vi "Calculator.vi"() -> ()   [LabVIEW 2020]
panel:
  in  "Operator":T1(ring)
  out "Result":dbl
  in  "Input B":dbl
  in  "Input A":dbl
  # "Simple Calculator"
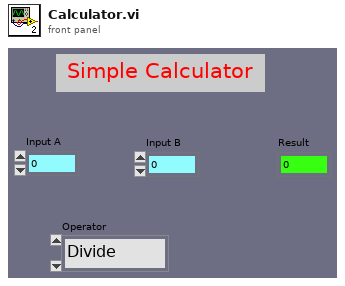
[diagram p1: front panel]
types:
  T1 = enum16{"Divide", "Multiply", "Add", "Subtract", ""}
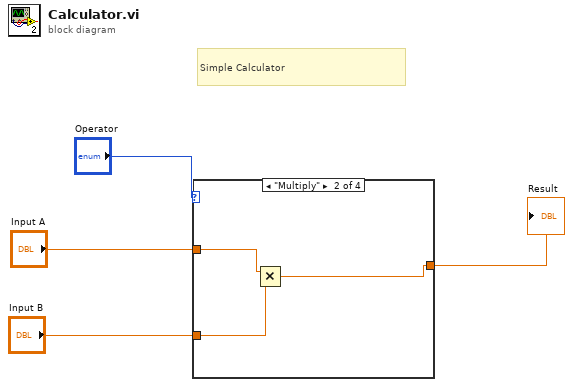
[diagram p0: block diagram]
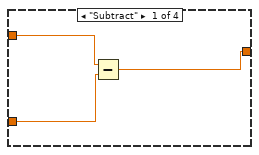
[diagram p2: hidden frame]
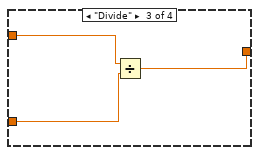
[diagram p3: hidden frame]
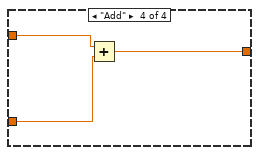
[diagram p4: hidden frame]
diagram:
  # "Simple Calculator"
  n1 = case shown="\"Multiply\"" "Operator" {
    tunnel: "Input A" -> [w7 w10 w13 w16]
    tunnel: "Input B" -> [w6 w9 w12 w15]
    tunnel: [w5 w8 w11 w14] -> w2
    frame "Subtract" {
      n2 = Subtract(x=w7, y=w6) -> (x-y=w5:dbl)
    }
    frame "Multiply" {
      n3 = Multiply(x=w10, y=w9) -> (x*y=w8:dbl)
    }
    frame "Divide" {
      n4 = Divide(x=w13, y=w12) -> (x/y=w11:dbl)
    }
    frame "Add" {
      n5 = Add(x=w16, y=w15) -> (x+y=w14:dbl)
    }
  }
  "Result" <- w2
